vi "Configure Verbosity.vi"(8 "Error In":errorcluster, 11 "Verbosity":u8=4) -> (0 "Error Out":errorcluster)   [LabVIEW 2015, in "Logger.lvlib"]
doc: "Sets the verbosity for displaying an error dialog to a user when using the Catch Error VI for error handling."
uses:
  Logger.lvlib
  Private/Error/Action.ctl
  Private/Error/Error.lvlib
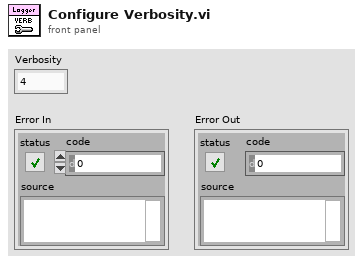
[diagram p1: front panel]
types:
  T1 = typedef "Logger.lvlib/Error.lvlib/Action.ctl" = enum16{"Initialize", "Get", "Set Verbosity", "Set User-Defined Codes", "Set User-Defined Descriptions", "Shutdown"}
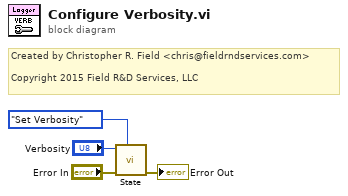
[diagram p0: block diagram]
diagram:
  # "Created by Christopher R. Field <chris@fieldrndservices.com>\n\nCopyright 2015 Field R&D Services, LLC"
  n1 = call "State.vi"("Action"=Action."Set Verbosity", "Error In"="Error In", "Set Value"="Verbosity") -> ("Error Out"=→"Error Out":errorcluster)  [unwired: 7 in, 1 out]
